vi "Destroy FFT Library.vi"(8 "Error In":errorcluster) -> (0 "Error Out":errorcluster)   [LabVIEW 2012, in "OpenCLV x64.lvlib"]
doc: "Destroys the FFT Library"
uses:
  OpenCLV x64.lvlib
  Error Checking/Add Error Functional Global.vi
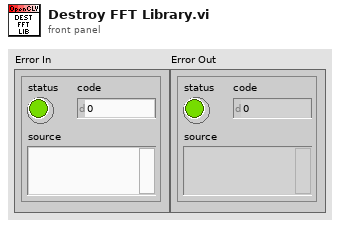
[diagram p1: front panel]
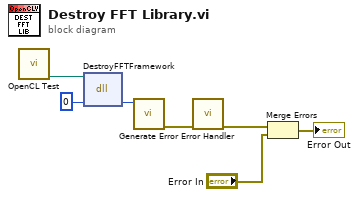
[diagram p0: block diagram]
diagram:
  n1 = call "OpenCL Test.vi"() -> ("DLL To Use"=w5:path)  [unwired: 11 in]
  n2 = dll-call lib="D:/OpenCLV/trunk/OpenCLV_x64_1.0/OpenCLV_x64d.dll" fn="DestroyFFTFramework"(path in=w5, "Error"=0) -> ("Error"=w6:i32)  [unwired: 3 in, 2 out]
  n3 = call "Generate Error.vi"("Error"=w6) -> ("error out"=w4:errorcluster)  [unwired: 10 in]
  n4 = call-poly "Error Handler.vi"("Error In"=w4) -> ("Error Out"=w3:errorcluster)  [unwired: 10 in]
  n5 = Merge Errors(w3, "Error In") -> (→"Error Out":errorcluster)
